vi "FGV_State.vi"(8 "errin":errorcluster, 10 "CMD":T1, 11 "State":enum16{"OFF", "PARK", "DRIVE", "LOAD"}(ring)) -> (0 "errout":errorcluster, 3 "Out":enum16{"OFF", "PARK", "DRIVE", "LOAD"}(ring))   [LabVIEW 2020]
uses:
  02 SLIM ZEN WS 500/SubVi/FGV.ctl
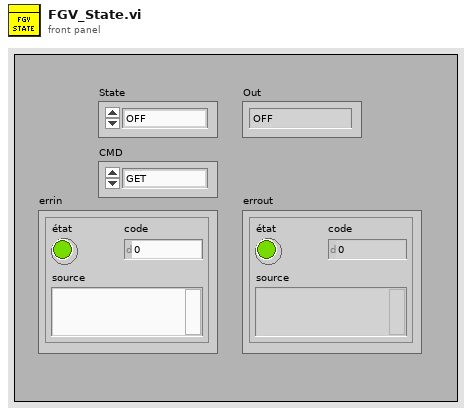
[diagram p1: front panel]
types:
  T1 = typedef "FGV.ctl" = enum16{"GET", "SET", "RAZ"}
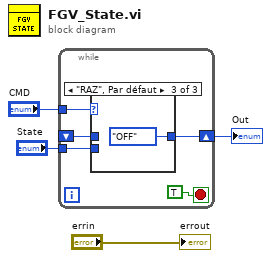
[diagram p0: block diagram]
diagram:
  n1 = while {
    tunnel: "CMD" -> [w8]
    shift-right: [w7] -> w3
    shift-left: _ -> [w6]
    tunnel: "State" -> [w5]
    stop <- TRUE stop-if-true
    n2 = case shown="\"RAZ\", Par défaut" w8 {
      tunnel: [w10 w11 enum16{"OFF", "PARK", "DRIVE", "LOAD"}."OFF" ("State")] -> w7
      tunnel: w6 -> [w10 _ _]
      tunnel: w5 -> [_ w11 _]
      frame "GET" {
      }
      frame "SET" {
      }
      frame "RAZ", Default {
      }
    }
  }
  "Out" <- w3
  "errout" <- "errin"
